vi "Create map.vi"(8 "error in (no error)":errorcluster, 11 "n (number of nodes on a side)":i32=3) -> (0 "error out":errorcluster, 1 "no. of columns":i32, 2 "no. of rows":i32, 3 "map\n2D array of nodes\n(n) x (n) size":T1[][](array[typedef]))   [LabVIEW 2021, in "Project Euler.lvlib"]
uses:
  Project Euler.lvlib
  lattice_path_node.ctl
  lattice_path_direction.ctl
panel:
  out "current j":i32
  out "current i":i32
  # "Development\ncontrols/indicators useful for development and testing, but which are not outputs of the VI"
  # "Input\nInputs to the VI"
  # "Output\nOutputs of the VI"
  # "Description\n\nBlank VI with error handling case. \n\nSummarize the use of this VI in this space."
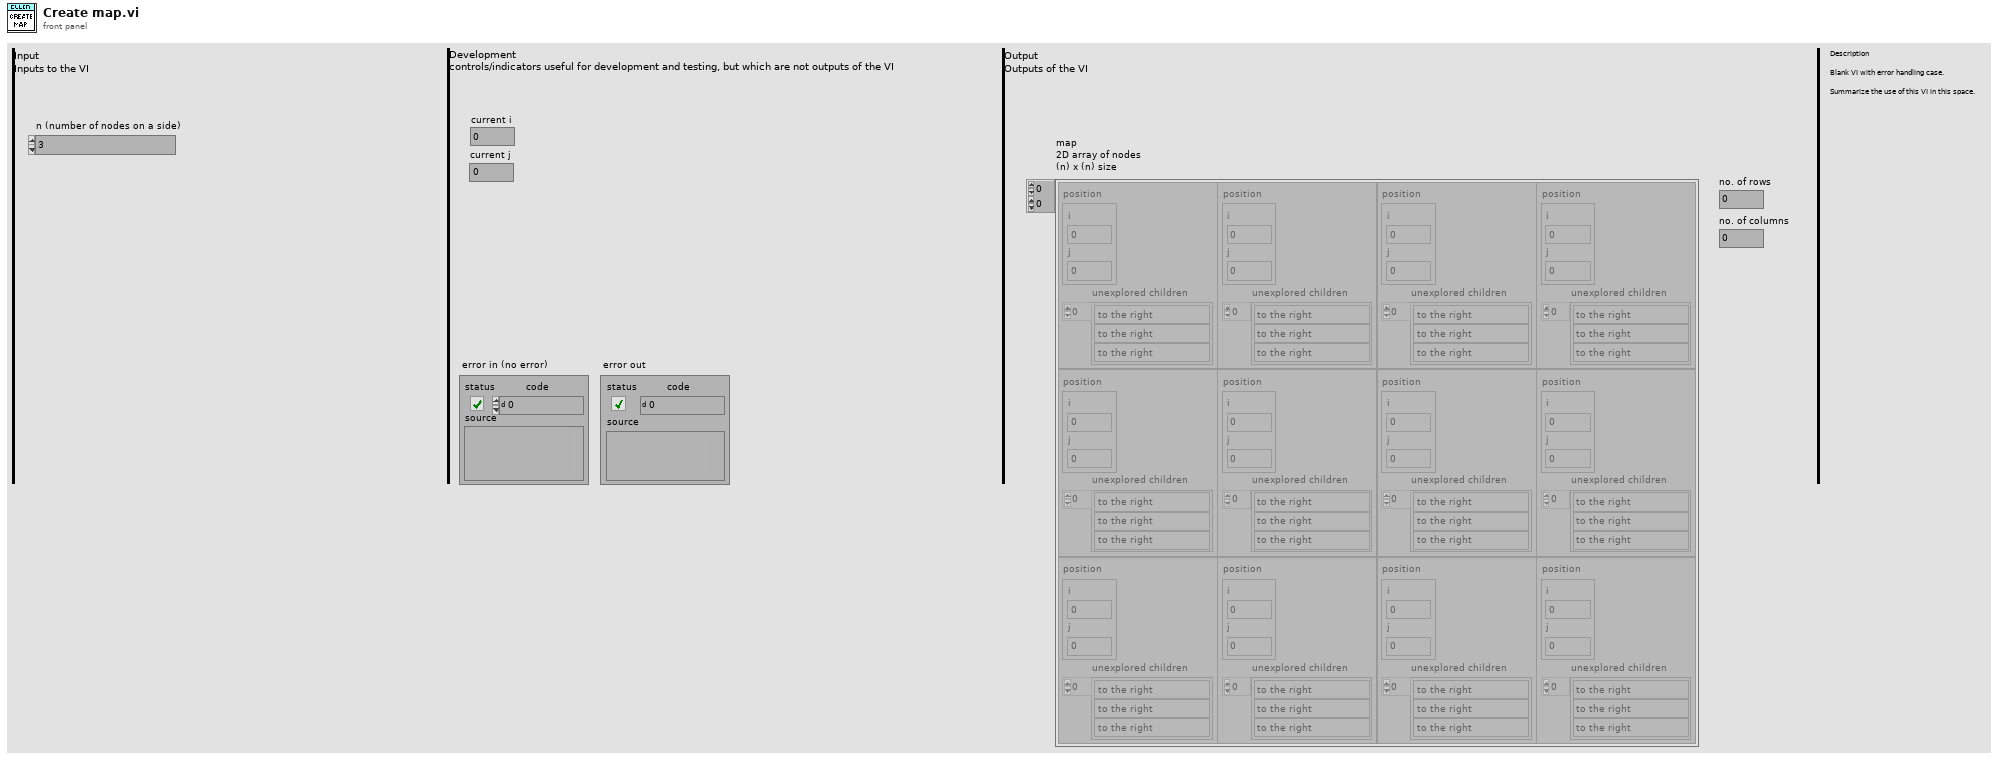
[diagram p1: front panel]
types:
  T1 = typedef "Project Euler.lvlib/lattice_path_node.ctl" = cluster{"position":cluster{"i":i32, "j":i32}, "unexplored children":T2[]}
  T2 = typedef "Project Euler.lvlib/lattice_path_direction.ctl" = enum16{"to the right", "downwards"}
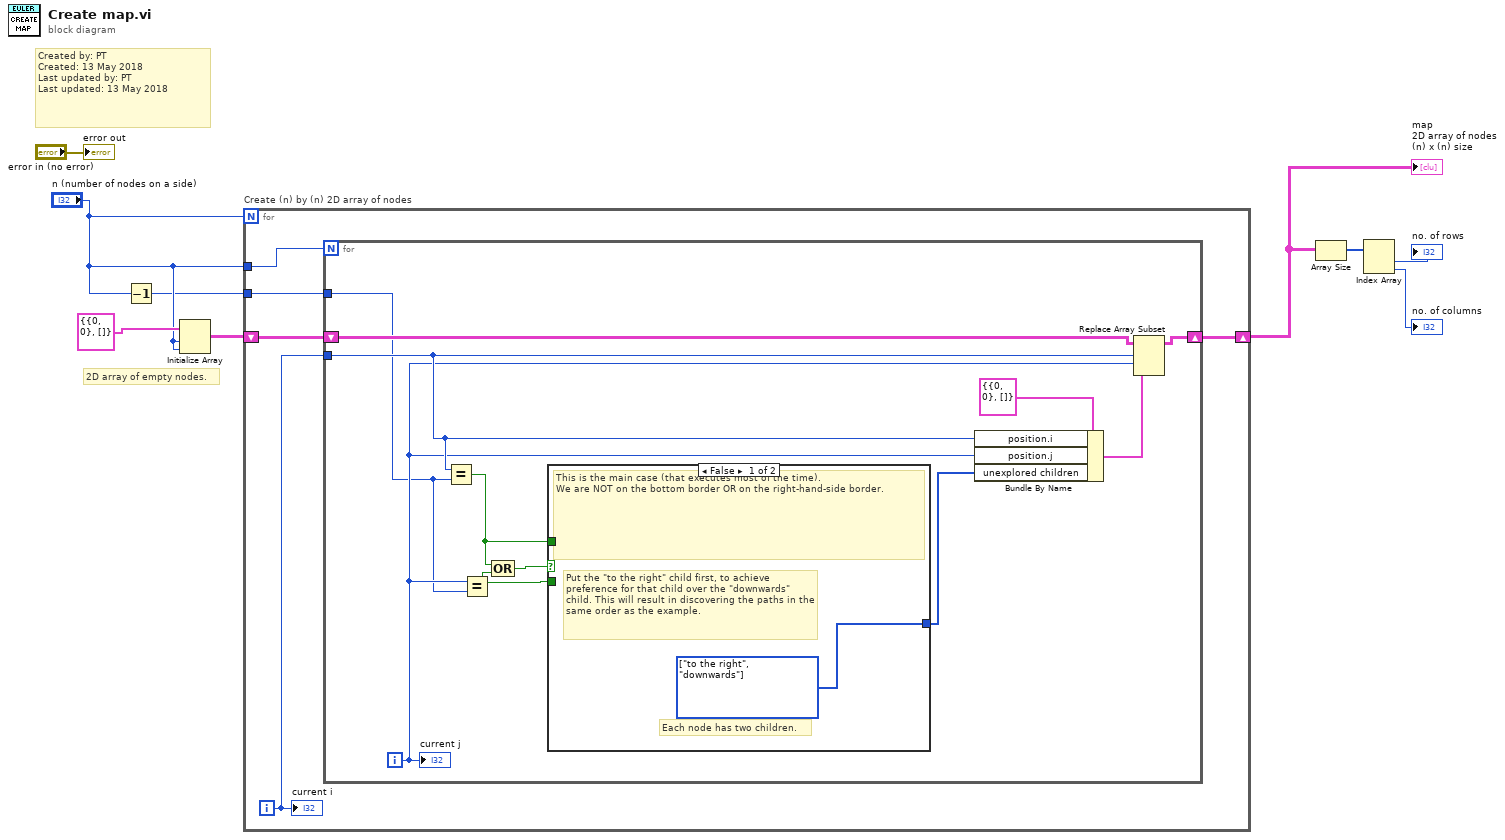
[diagram p0: block diagram]
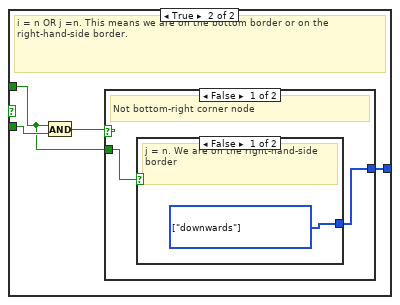
[diagram p2: hidden frame]
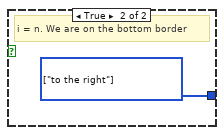
[diagram p3: hidden frame]
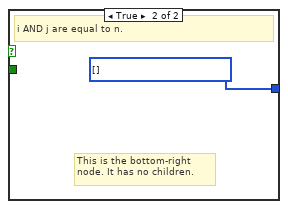
[diagram p4: hidden frame]
diagram:
  # "2D array of empty nodes."
  # "Created by: PT\nCreated: 13 May 2018\nLast updated by: PT\nLast updated: 13 May 2018"
  n1 = Decrement(x="n (number of nodes on a side)") -> (x-1=w1:i32)
  n2 = Initialize Array(T1 {"position"={"i"=0, "j"=0}, "unexplored children"=[]} ("node"), "n (number of nodes on a side)", "n (number of nodes on a side)") -> (w7:T1[][])
  n3 = for "Create (n) by (n) 2D array of nodes" {
    N: "n (number of nodes on a side)" -> [_]
    tunnel: "n (number of nodes on a side)" -> [w14]
    shift-right: [w11] -> w2
    shift-left: w7 -> [w13]
    tunnel: w1 -> [w10]
    i -> [w12]
    n4 = for {
      N: w14 -> [_]
      tunnel: w12 -> [w21]
      shift-right: [w22] -> w11
      shift-left: w13 -> [w25]
      tunnel: w10 -> [w19]
      i -> [w20]
      n5 = Equal?(x=w21, y=w19) -> (x = y?=w16:bool)
      n6 = Equal?(x=w20, y=w19) -> (x = y?=w15:bool)
      n7 = Compound Arithmetic op=OR(w16, w15) -> (w18:bool)
      n8 = case shown="False" w18 {
        tunnel: [w26 w28] -> w17
        tunnel: w16 -> [_ w27]
        tunnel: w15 -> [_ w30]
        frame False {
          w26 = T2[] [enum."to the right", enum."downwards"] items=["to the right", "downwards"] ("children")
          # "Put the \"to the right\" child first, to achieve preference for that child over the \"downwards\" child. This will result in discovering the paths in the same order as the example."
          # "Each node has two children."
          # "This is the main case (that executes most of the time).\nWe are NOT on the bottom border OR on the right-hand-side border."
        }
        frame True {
          # "i = n OR j =n. This means we are on the bottom border or on the right-hand-side border."
          n9 = And(x=w27, y=w30) -> (x .and. y?=w29:bool)
          n10 = case shown="False" w29 {
            tunnel: [w31 w35] -> w28
            tunnel: w27 -> [w32 _]
            frame False {
              # "Not bottom-right corner node"
              n11 = case shown="False" w32 {
                tunnel: [w33 w34] -> w31
                frame False {
                  w33 = T2[] [enum."downwards"] items=["to the right", "downwards"] ("children")
                  # "j = n. We are on the right-hand-side border"
                }
                frame True {
                  w34 = T2[] [enum."to the right"] items=["to the right", "downwards"] ("children")
                  # "i = n. We are on the bottom border"
                }
              }
            }
            frame True {
              w35 = T2[] [] items=["to the right", "downwards"] ("children")
              # "This is the bottom-right node. It has no children."
              # "i AND j are equal to n."
            }
          }
        }
      }
      n12 = Bundle By Name(cluster=T1 {"position"={"i"=0, "j"=0}, "unexplored children"=[]} ("node"), "position.i"=w21, "position.j"=w20, "unexplored children"=w17) -> (w23:T1)
      n13 = Replace Array Subset(array=w25, new element=w23, index (row)=w21, index (col)=w20) -> (w22:T1[][])
      "current j" <- w20
    }
    "current i" <- w12
  }
  "map\n2D array of nodes\n(n) x (n) size" <- w2
  n14 = Array Size(array=w2) -> (size(s)=w5:i32[])
  n15 = Index Array(array=w5) -> (element #1=→"no. of rows":i32, element #2=→"no. of columns":i32)  [unwired: 2 in]
  "error out" <- "error in (no error)"
